vi "CSM - Wait for All Modules to be Alive.vi"(6 "Timeout(5000ms)":u32=5000, 8 "Error in":errorcluster caption="Error in (no error)", 11 "Module Names (in)":string[](array[string])) -> (0 "Error out":errorcluster, 1 "waited(ms)":u32, 2 "Left Modules":string[](array[string]))   [LabVIEW 2020, in "Communicable State Machine.lvlib"]
doc: "List all CSM Modules alive in system.\n\n<b>Inputs:</b>\n - <b>Exclude Standalone CSM(T)</b>: 'TRUE' to exclude standalone CSM module, and 'FALSE' to include them.\n - <b>Error in</b>: Error cluster\n\n<b>Outputs:</b>\n - <b>Module Names</b>: Module Names\n - <b>Error out</b>: Error cluster"
uses:
  Communicable State Machine.lvlib
  global-CSMQ FGV Change Flag.vi
  _CSMOFGV.vi
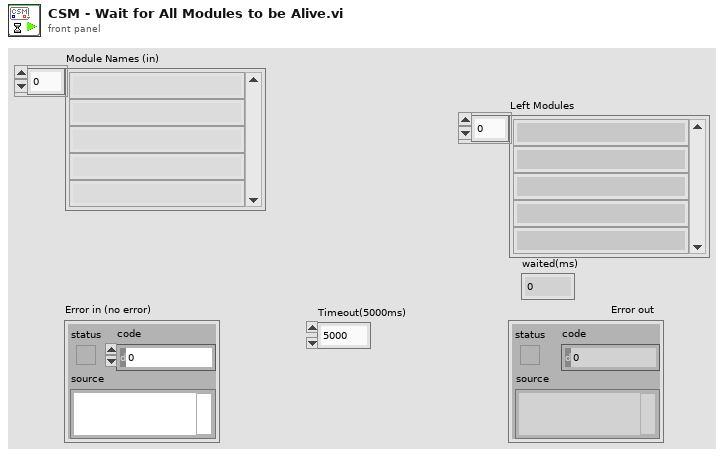
[diagram p1: front panel]
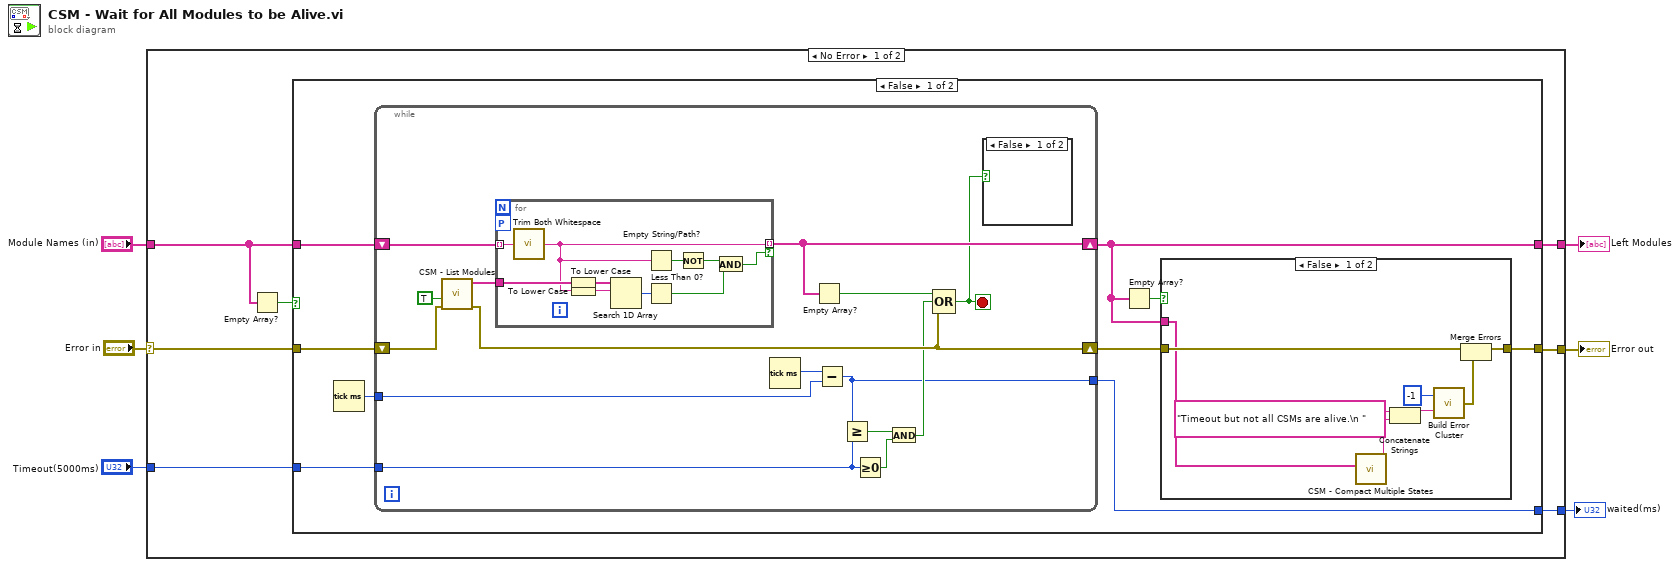
[diagram p0: block diagram]
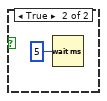
[diagram p3: hidden frame]
diagram:
  n1 = case shown="No Error" "Error in" {
    selector: "Error in" -> [w13 w61]
    tunnel: [w11 w61] -> w5
    tunnel: "Module Names (in)" -> [w8 w60]
    tunnel: [w10 w60] -> w3
    tunnel: "Timeout(5000ms)" -> [w12 _]
    tunnel: [w7 _] -> w1
    frame No Error {
      n2 = Empty Array?(array=w8) -> (empty?=w9:bool)
      n3 = case shown="False" w9 {
        tunnel: w8 -> [w22 w59]
        tunnel: w13 -> [w21 w58]
        tunnel: w12 -> [w19 _]
        tunnel: [w17 w58] -> w11
        tunnel: [w15 w59] -> w10
        tunnel: [w14 _] -> w7
        frame False {
          n4 = Tick Count (ms)() -> (millisecond timer value=w20:u32)
          n5 = while {
            shift-right: [w43] -> w15
            shift-left: w22 -> [w45]
            shift-right: [w40] -> w16
            shift-left: w21 -> [w42]
            tunnel: w20 -> [w39]
            tunnel: w19 -> [w37]
            tunnel: [w32] -> w14
            stop <- w38 stop-if-true
            n6 = call "CSM - List Modules.vi"("Error in"=w42, "All?"=TRUE) -> ("Error out"=w40:errorcluster, "Module Names"=w44:string[])  [unwired: 8 in]
            n7 = for {
              tunnel: w45 -> [w53] mode=indexing
              tunnel: w44 -> [w57]
              tunnel: [w49] -> w43 mode=indexing if=w51
              workers-P: _ -> [_]
              n8 = call "Trim Both Whitespace.vi"("string"=w53) -> ("trimmed string"=w49:string)  [unwired: 1 in]
              n9 = To Lower Case(string=w57) -> (all lower case string=w55:string[])
              n10 = To Lower Case(string=w49) -> (all lower case string=w54:string)
              n11 = Search 1D Array(1D array=w55, element=w54) -> (index of element=w56:i32)  [unwired: 1 in]
              n12 = Empty String/Path?(string/path=w49) -> (empty?=w50:bool)
              n13 = Less Than 0?(x=w56) -> (x < 0?=w52:bool)
              n14 = Not(x=w50) -> (.not. x?=w48:bool)
              n15 = And(x=w48, y=w52) -> (x .and. y?=w51:bool)
            }
            n16 = Tick Count (ms)() -> (millisecond timer value=w36:u32)
            n17 = Empty Array?(array=w43) -> (empty?=w41:bool)
            n18 = Subtract(x=w36, y=w39) -> (x-y=w32:u32)
            n19 = Greater Or Equal?(x=w32, y=w37) -> (x >= y?=w34:bool)
            n20 = Greater Or Equal To 0?(x=w37) -> (x >= 0?=w33:bool)
            n21 = And(x=w34, y=w33) -> (x .and. y?=w35:bool)
            n22 = Compound Arithmetic op=OR(w41, w35, w40) -> (w38:bool)
            n23 = case shown="False" w38 {
              frame False {
              }
              frame True {
                n24 = Wait (ms)(milliseconds to wait=u32 5) -> ()  [unwired: 1 out]
              }
            }
          }
          n25 = Empty Array?(array=w15) -> (empty?=w18:bool)
          n26 = case shown="False" w18 {
            tunnel: [w29 w31] -> w17
            tunnel: w16 -> [w30 w31]
            tunnel: w15 -> [w24 _]
            frame False {
              n27 = call "CSM - Compact Multiple States.vi"("Multiple States"=w24) -> ("States"=w23:string)  [unwired: 9 in]
              n28 = Concatenate Strings("Timeout but not all CSMs are alive.\n " ("String to Prepend to source (\"\")"), w23) -> (w25:string)
              n29 = call "Build Error Cluster.vi"("String to Prepend to source (\"\")"=w25, "code"=-1) -> ("error out"=w28:errorcluster)
              n30 = Merge Errors(w30, w28) -> (w29:errorcluster)
            }
            frame True {
            }
          }
        }
        frame True {
        }
      }
    }
    frame Error {
    }
  }
  "Error out" <- w5
  "Left Modules" <- w3
  "waited(ms)" <- w1
